vi "GEA2 Read Message.vi"(0 "GEA2 Reference In":refnum<k24>, 1 "Expected Source":string=".*", 5 "Expected Command":string=".*", 7 "Expected Data":string=".*", 9 "Timeout (ms)":u32=500, 11 "Error In":errorcluster, 12 "# of Tries":u8=5 min=1) -> (4 "GEA2 Reference Out":refnum<k24>, 6 "Raw Data Out":string, 8 "Coverted Data Out":T1 {"CRC" format="%04x"; "Length" format="%02x"; "Command" format="%02x"; "Destination" format="%02x"; "Source" format="%02x"}, 15 "Error Out":errorcluster)   [LabVIEW 2018, in "GEA2_Toolkit.lvlib"]
doc: "This VI listens on the bus for a specified timeout until the expected command / data is returned."
uses:
  C:/Users/iallatyp/Desktop/New folder/GEA3/library/GEA2_Toolkit.lvlib
  D:/Common/LabVIEW GEA2 Toolkit/source/GEA3 DLL Source/GeaCommunication.dll
  source/GEA3 DLL Source/GeaCommunication.dll
  type defs/Data Out.ctl
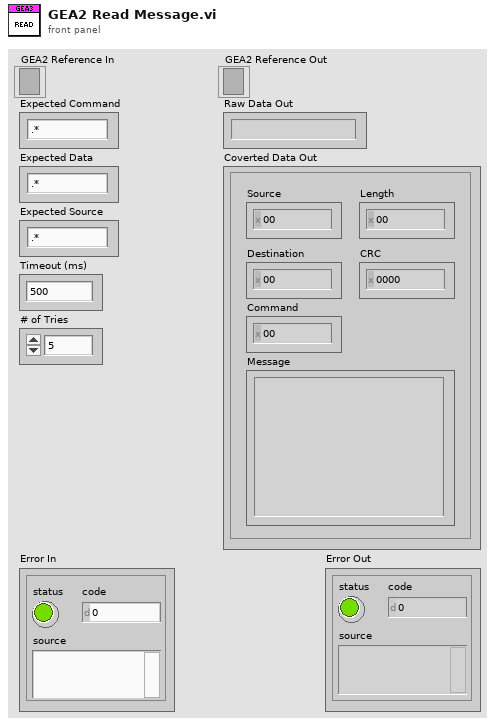
[diagram p1: front panel]
types:
  T1 = typedef "GEA2_Toolkit.lvlib/Data Out.ctl" = cluster{"Source":u8, "Destination":u8, "Command":u8, "Length":u8, "CRC":u16, "Message":string}
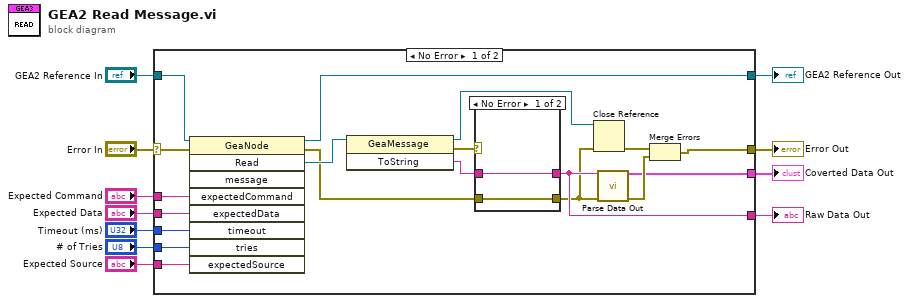
[diagram p0: block diagram]
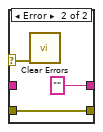
[diagram p2: hidden frame]
diagram:
  n1 = case shown="No Error" "Error In" {
    selector: "Error In" -> [w25 w36]
    tunnel: "GEA2 Reference In" -> [w29 w37]
    tunnel: [w24 w37] -> w8
    tunnel: [w18 w36] -> w10
    tunnel: "Expected Command" -> [w28 _]
    tunnel: "Expected Data" -> [w27 _]
    tunnel: "Timeout (ms)" -> [w26 _]
    tunnel: [w17 _] -> w4
    tunnel: [w16 _] -> w3
    tunnel: "# of Tries" -> [w13 _]
    tunnel: "Expected Source" -> [w12 _]
    frame No Error {
      n2 = invoke class="GeaNode" method="Read"(reference=w29, error in=w25, "expectedCommand"=w28, "expectedData"=w27, "timeout"=w26, "tries"=w13, "expectedSource"=w12) -> (reference out=w24:refnum<k24>, error out=w14:errorcluster, "Read"=w30:refnum<k24>)  [unwired: 2 in, 6 out]
      n3 = invoke class="GeaMessage" method="ToString"(reference=w30) -> (reference out=w21:refnum<k24>, error out=w22:errorcluster, "ToString"=w23:string)  [unwired: 2 in]
      n4 = case shown="No Error" w22 {
        selector: w22 -> [_ w34]
        tunnel: w23 -> [w32 _]
        tunnel: [w32 "" ("ToString")] -> w17
        tunnel: [w31 w33] -> w15
        tunnel: w14 -> [w31 w33]
        frame No Error {
        }
        frame Error {
          n5 = call <vilib>:"Clear Errors.vi"("error in (no error)"=w34) -> ()  [unwired: 5 in, 2 out]
        }
      }
      n6 = Close Reference(reference=w21, error in (no error)=w15) -> (error out=w20:errorcluster)
      n7 = call "Parse Data Out.vi"("Raw Data In"=w17, "Error In"=w15) -> ("Data Out"=w16:T1, "Error Out"=w19:errorcluster)  [unwired: 11 in, 1 out]
      n8 = Merge Errors(w20, w19) -> (w18:errorcluster)
    }
    frame Error {
    }
  }
  "Error Out" <- w10
  "GEA2 Reference Out" <- w8
  "Raw Data Out" <- w4
  "Coverted Data Out" <- w3
